vi "Inverter Process Core.vi"() -> ()   [LabVIEW 2019, in "Main.lvclass"]
uses:
  Main.lvclass
  DataTypes/PrivateAsynEv_Main--enum.ctl
  Common/DataTypes/Measurement Config--cluster.ctl
  Common/DataTypes/Acquisition Mode--cluster.ctl
  Common/DataTypes/DAQState--enum.ctl
  Common/DataTypes/LogState--enum.ctl
  Common/DataTypes/TDMSState--enum.ctl
  DataTypes/ProcessingState--enum.ctl
  Common/DataTypes/inverter offset range--cluster.ctl
  Common/DataTypes/inverter gain range--cluster.ctl
  Common/DataTypes/inverter info v2--cluster.ctl
  Common/DataTypes/Inverter database record v2--cluster.ctl
  support/Data Algorithms/subvis/DataTypes/ESR alarm variables.ctl
  support/Data Algorithms/subvis/DataTypes/averaging variables.ctl
  support/Data Algorithms/subvis/DataTypes/Processing loop variables--cluster.ctl
  Common/DataTypes/RawChannelData--cluster.ctl
  Common/DataTypes/RawDAQData--cluster.ctl
  support/Data Algorithms/subvis/DataTypes/Gain control.ctl
  support/Data Algorithms/subvis/DataTypes/ESR scaling--cluster.ctl
  Common/DataTypes/TD Async CmdMsg EventData--cluster.ctl
  Common/DataTypes/UpdateControlValue EvData--cluster.ctl
  DataTypes/ProcessingStateChg EvData--cluster.ctl
  DataTypes/Public Events--cluster.ctl
  DAQ_Engine/DAQ_Engine.lvclass
  Config/Config.lvclass
  Log_Engine/Log_Engine.lvclass
  DataTypes/Dependency--cluster.ctl
  DataTypes/Settings--cluster.ctl
  Common/DataTypes/RawDAQDataQRef--cluster.ctl
  Common/DataTypes/ChannelWaveforms--cluster.ctl
  Common/DataTypes/InverterWaveforms--cluster.ctl
  Common/DataTypes/InverterWaveforms--QRef.ctl
  DataTypes/DataProcessAuxData--cluster.ctl
  Common/DataTypes/DataProcAuxDat--Qref.ctl
  DataTypes/InverterInfo--cluster.ctl
  DataTypes/Process - AppData--cluster.ctl
panel:
  in  "SM2 AppData":T1={"Core"={"Current VI Reference"=refnum, "Close Panel on Exit?"=FALSE}, "Your Boolean data"=FALSE, "Your string data"="", "SMQ"=refnum, "Initialized?"=FALSE, "Self Reference"=refnum, "Simulation?"=FALSE, "process sync"=refnum, "vData"=variant, "Settings"={"Simulation"=FALSE, "Signal scaling"=[], "ESR scaling"=[], "num readings to average"=[], "ESR alarm threshhold (%)"=[], "UseDummyVrms"=FALSE, "Dummy Vrms"=0.0, "Inverter Database File"=path "", "default Inverter (name)"=[]}, "Dependency"={"Config"=refnum, "DAQ"=refnum, "Log_Engine"=refnum}, "Public Events"={"Main.AsyncCmd Event"=refnum, "Main.AsyncMsg Event"=refnum, "stop process"=refnum, "UpdateControlValue Ev"=refnum, "ProcessingStateChg Ev"=refnum}, "RawDaqDataQ"=refnum, "InverterWaveformsQ"=refnum, "Processing loop variables"={"DUT ESR avg"=[], "DUT  PF avg"=[], "DUT  Power avg "=[], "DUT processed data"=[], "ESR alarm variables"=[], "Status data"=[], "CurrInverter"=[], "miscellaneous"=[], "DUT INVERTER data"=[]}, "Measurement config"={"Data Rate 9775"=3.0, "Data Rate 9215"=1200000.0, "Samples RMS 9215"=480000, "Samples RMS 9775"=3}, "Acquisition mode"=enum."3phase", "DAQState"=enum."Unknown", "Signal scaling"={"Iin ripple gain"=13.333, "Iout ripple gain"=13.333, "Iout 60Hz gain "=14.286, "Vout 60Hz gain "=20.0, "Iin ripple offest"=0.0, "Iout ripple offset"=0.0, "Iout 60Hz offset"=0.0, "Vout 60Hz offset"=0.0}, "PrivateAsync Ev"=refnum, "LogState"=enum."Unknown", "TDMSState"=enum."Unknown", "InvWfmsQ-DT"=refnum, "DPAuxDataQ"=refnum, "ProcessingState"=enum."Idle", "InverterInfo"={"Inverter ID"=""}, "ProcLoopInterval"=0, "StoredESR Baseline"=[], "StoreESR BLine Flag"=FALSE, "UseSavedESR BLine Flag"=FALSE} {"Processing loop variables"."CurrInverter"."last updated" format="%<%H:%M\n%d/%m/%Y>T"; "Processing loop variables"."CurrInverter"."set flag" items=["False", "True"]; "Settings"."Dummy Vrms" format="%.2g"}
  in  "ESR scaling":T4
  in  "UseDummyVrms":bool
  in  "Dummy Vrms":dbl=120.0
  in  "reset averaging":bool
  in  "Signal scaling":T3={"Iin ripple gain"=13.333, "Iout ripple gain"=13.333, "Iout 60Hz gain "=14.286, "Vout 60Hz gain "=20.0, "Iin ripple offest"=0.0, "Iout ripple offset"=0.0, "Iout 60Hz offset"=0.0, "Vout 60Hz offset"=0.0}
  out "DAQ data":T24
  out "RawDaqDataQ size":i32
  in  "sampling rate (Hz)":i32
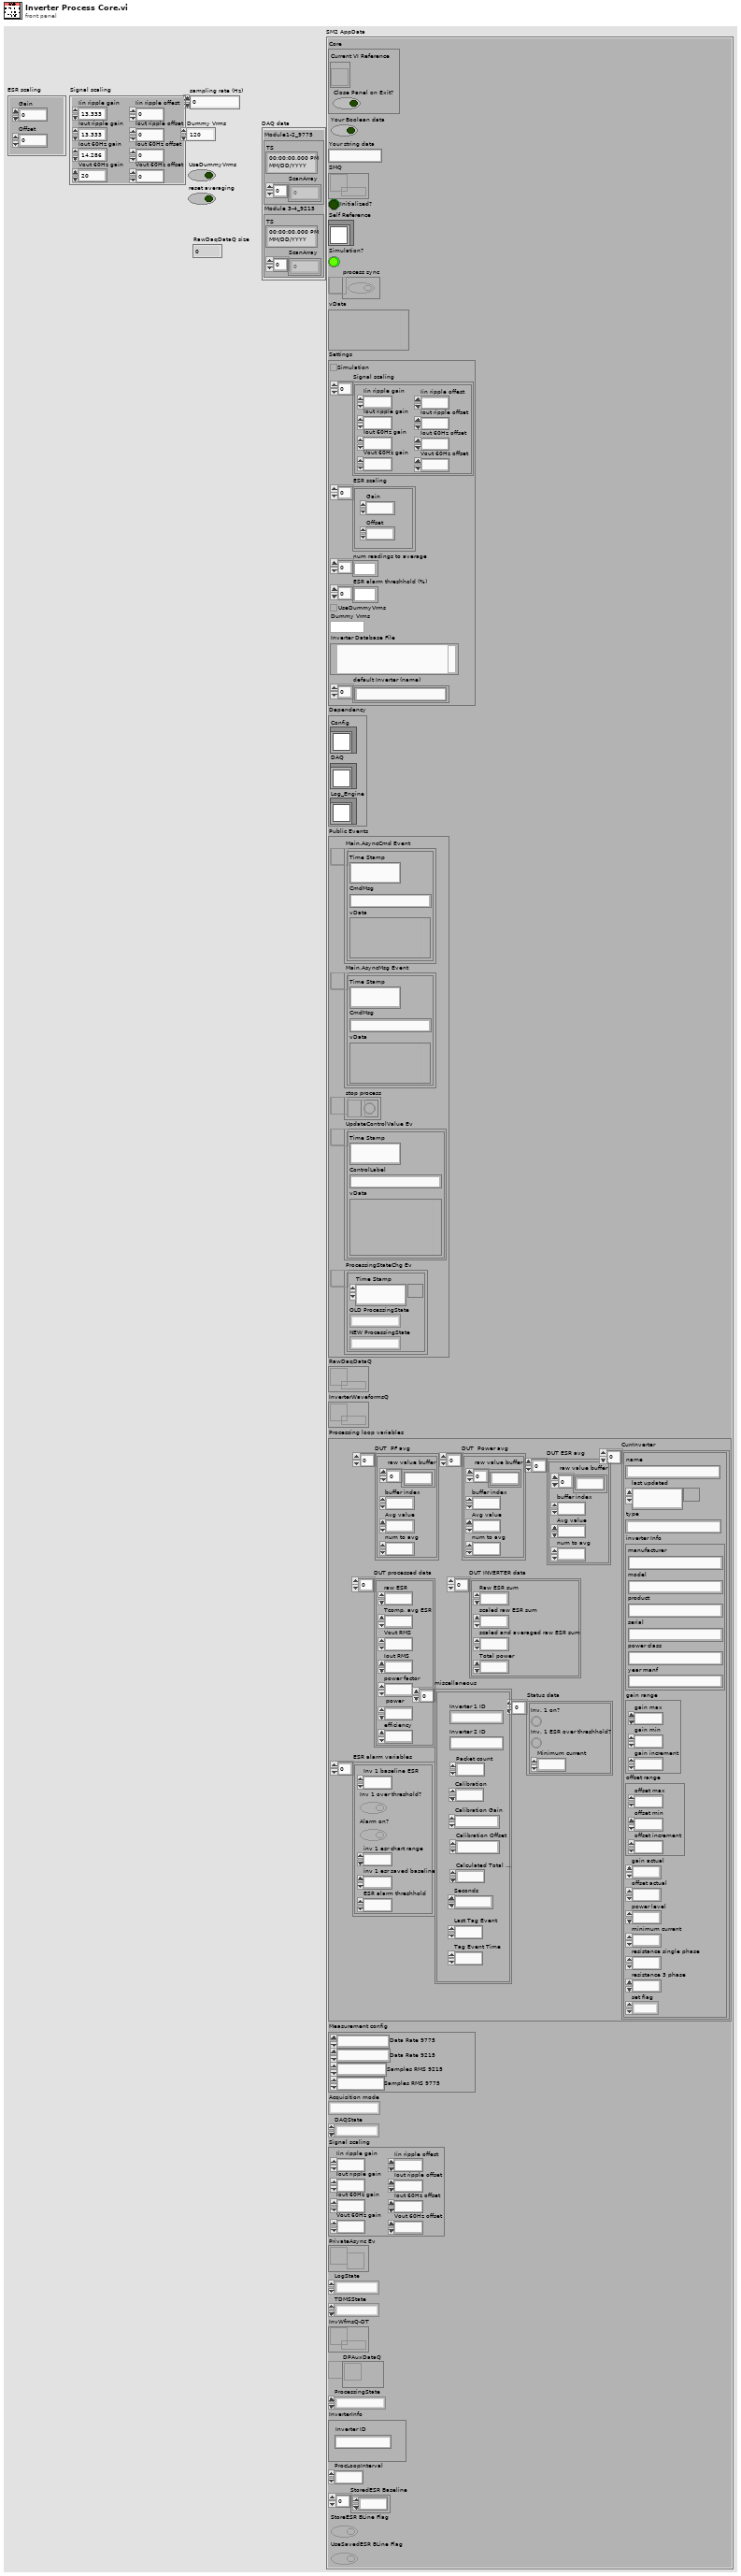
[diagram p1: front panel]
types:
  T1 = typedef "Main.lvclass/Process - AppData--cluster.ctl" = cluster{"Core":cluster{"Current VI Reference":refnum<vi>, "Close Panel on Exit?":bool}, "Your Boolean data":bool, "Your string data":string, "SMQ":refnum<queue>, "Initialized?":bool, "Self Reference":refnum<class "Main.lvclass">, "Simulation?":bool, "process sync":refnum<notifier>, "vData":variant, "Settings":T2, "Dependency":T5, "Public Events":T6, "RawDaqDataQ":T7, "InverterWaveformsQ":T8, "Processing loop variables":T9, "Measurement config":T16, "Acquisition mode":T17, "DAQState":T18, "Signal scaling":T3, "PrivateAsync Ev":refnum<user-event>, "LogState":T19, "TDMSState":T20, "InvWfmsQ-DT":T8, "DPAuxDataQ":T21, "ProcessingState":T22, "InverterInfo":T23, "ProcLoopInterval":u32, "StoredESR Baseline":dbl[], "StoreESR BLine Flag":bool, "UseSavedESR BLine Flag":bool}
  T2 = typedef "Main.lvclass/Settings--cluster.ctl" = cluster{"Simulation":bool, "Signal scaling":T3[], "ESR scaling":T4[], "num readings to average":i32[], "ESR alarm threshhold (%)":i32[], "UseDummyVrms":bool, "Dummy Vrms":dbl, "Inverter Database File":path, "default Inverter (name)":string[]}
  T3 = typedef "Main.lvclass/Gain control.ctl" = cluster{"Iin ripple gain":dbl, "Iout ripple gain":dbl, "Iout 60Hz gain ":dbl, "Vout 60Hz gain ":dbl, "Iin ripple offest":dbl, "Iout ripple offset":dbl, "Iout 60Hz offset":dbl, "Vout 60Hz offset":dbl}
  T4 = typedef "Main.lvclass/ESR scaling--cluster.ctl" = cluster{"Gain":dbl, "Offset":dbl}
  T5 = typedef "Main.lvclass/Dependency--cluster.ctl" = cluster{"Config":refnum<class "Config.lvclass">, "DAQ":refnum<class "DAQ_Engine.lvclass">, "Log_Engine":refnum<class "Log_Engine.lvclass">}
  T6 = typedef "Main.lvclass/Public Events--cluster.ctl" = cluster{"Main.AsyncCmd Event":refnum<user-event>, "Main.AsyncMsg Event":refnum<user-event>, "stop process":refnum<user-event>, "UpdateControlValue Ev":refnum<user-event>, "ProcessingStateChg Ev":refnum<user-event>}
  T7 = typedef "RawDAQDataQRef--cluster.ctl" = refnum<queue>
  T8 = typedef "InverterWaveforms--QRef.ctl" = refnum<queue>
  T9 = typedef "Main.lvclass/Processing loop variables--cluster.ctl" = cluster{"DUT ESR avg":T10[], "DUT  PF avg":T10[], "DUT  Power avg ":T10[], "DUT processed data":cluster{"raw ESR":dbl, "Tcomp, avg ESR":dbl, "Vout RMS":dbl, "Iout RMS":dbl, "power factor":dbl, "power":dbl, "efficiency":dbl}[], "ESR alarm variables":T11[], "Status data":cluster{"Inv. 1 on?":bool, "Inv. 1 ESR over threshhold?":bool, "Minimum current":dbl}[], "CurrInverter":T12[], "miscellaneous":cluster{"Inverter 1 ID":string, "Inverter 2 ID":string, "Packet count":u32, "Calibration":dbl, "Calibration Gain":dbl, "Calibration Offset":dbl, "Calculated Total Power":dbl, "Seconds":dbl, "Last Tag Event":dbl, "Tag Event Time":dbl}[], "DUT INVERTER data":cluster{"Raw ESR sum":dbl, "scaled raw ESR sum":dbl, "scaled and averaged raw ESR sum":dbl, "Total power":dbl}[]}
  T10 = typedef "Main.lvclass/averaging variables.ctl" = cluster{"raw value buffer":dbl[], "buffer index":i32, "Avg value":dbl, "num to avg":i32}
  T11 = typedef "Main.lvclass/ESR alarm variables.ctl" = cluster{"Inv 1 baseline ESR":dbl, "Inv 1 over threshold?":bool, "Alarm on?":bool, "inv 1 esr chart range":dbl, "inv 1 esr saved baseline":dbl, "ESR alarm threshhold":dbl}
  T12 = typedef "Inverter database record v2--cluster.ctl" = cluster{"name":string, "last updated":timestamp, "type":string, "inverter Info":T13, "gain range":T14, "offset range":T15, "gain actual":dbl, "offset actual":dbl, "power level":dbl, "minimum current":dbl, "resistance single phase":dbl, "resistance 3 phase":dbl, "set flag":u16}
  T13 = typedef "inverter info v2--cluster.ctl" = cluster{"manufacturer":string, "model":string, "product":string, "serial":string, "power class":string, "year manf":string}
  T14 = typedef "inverter gain range--cluster.ctl" = cluster{"gain max":dbl, "gain min":dbl, "gain increment":dbl}
  T15 = typedef "inverter offset range--cluster.ctl" = cluster{"offset max":dbl, "offset min":dbl, "offset increment":dbl}
  T16 = typedef "Measurement Config--cluster.ctl" = cluster{"Data Rate 9775":dbl, "Data Rate 9215":dbl, "Samples RMS 9215":u32, "Samples RMS 9775":u32}
  T17 = typedef "Acquisition Mode--cluster.ctl" = enum16{"3phase", "Single"}
  T18 = typedef "DAQState--enum.ctl" = enum16{"Unknown", "Stopped", "Running", "Error"}
  T19 = typedef "LogState--enum.ctl" = enum16{"Unknown", "Stopped", "Running", "Error"}
  T20 = typedef "TDMSState--enum.ctl" = enum16{"Unknown", "Stopped", "Running", "Error"}
  T21 = typedef "DataProcAuxDat--Qref.ctl" = refnum<queue>
  T22 = typedef "Main.lvclass/ProcessingState--enum.ctl" = enum16{"Idle", "Starting", "Running", "Done", "Error"}
  T23 = typedef "InverterInfo--cluster.ctl" = cluster{"Inverter ID":string}
  T24 = typedef "RawDAQData--cluster.ctl" = cluster{"Module1-2_9775":T25, "Module 3-4_9215":T25}
  T25 = typedef "RawChannelData--cluster.ctl" = cluster{"TS":timestamp, "ScanArray":dbl[]}
  T26 = enum16{"Event Loop -", "Async Loop -", "DataProc Loop - "}
  T27 = typedef "Main.lvclass/PrivateAsynEv_Main--enum.ctl" = enum16{"PrivMain.UpdateMeasSettings", "PrivMain.UpdateAcqMode", "PrivMain.UpdateDAQState", "PrivMain.UpdateLogState", "PrivMain.UpdateTDMSState", "PrivMain.UpdateProcessingState", "PrivMain.Stop&Terminate", "PrivMain.CurrInverterUpdated", "PrivMain.UpdateStoreUseESRBaseline", "PrivMain.SetUnsetAlarm&ESRBLine", "PrivMain.ResetAveraging"}
  T28 = cluster{"VoltageDyn":dbl, "CurrentDyn":dbl, "MotorV SP":dbl}[]
  T29 = typedef "InverterWaveforms--cluster.ctl" = T30[]
  T30 = typedef "ChannelWaveforms--cluster.ctl" = cluster{"Iin ripple ":waveform(dbl), "Iout ripple ":waveform(dbl), "Iout 60Hz":waveform(dbl), "Vout 60Hz":waveform(dbl)}
  T31 = typedef "DataProcessAuxData--cluster.ctl" = cluster{"Time Stamp":timestamp, "Raw ESR sum":dbl, "Inv 1 ON?":bool, "Average scaled ESR sum":dbl, "Inv 1 over threshold?":bool, "Inv 1 ESR":cluster{"ESR Baseline":dbl, "Alarm threshhold (%)":dbl, "Avg value":dbl}, "Max ESR":dbl}
  T32 = typedef "TD MeasData--cluster.ctl" = cluster{"Timestamp":timestamp, "ESR_Ohm":dbl[], "DUT data":T33[], "DUT INVERTER data":cluster{"Raw ESR sum":dbl, "scaled raw ESR sum":dbl, "scaled and averaged raw ESR sum":dbl, "Total power":dbl}[]}
  T33 = typedef "InverterPhaseData--cluster.ctl" = cluster{"RawESR_Ohm":dbl, "TcompAvgESR_Ohm":dbl, "VoutRMS_V":dbl, "IoutRMS_A":dbl, "PF":dbl, "AvgPF":dbl, "Power_W":dbl, "AvgPower_W":dbl, "efficiency":dbl}
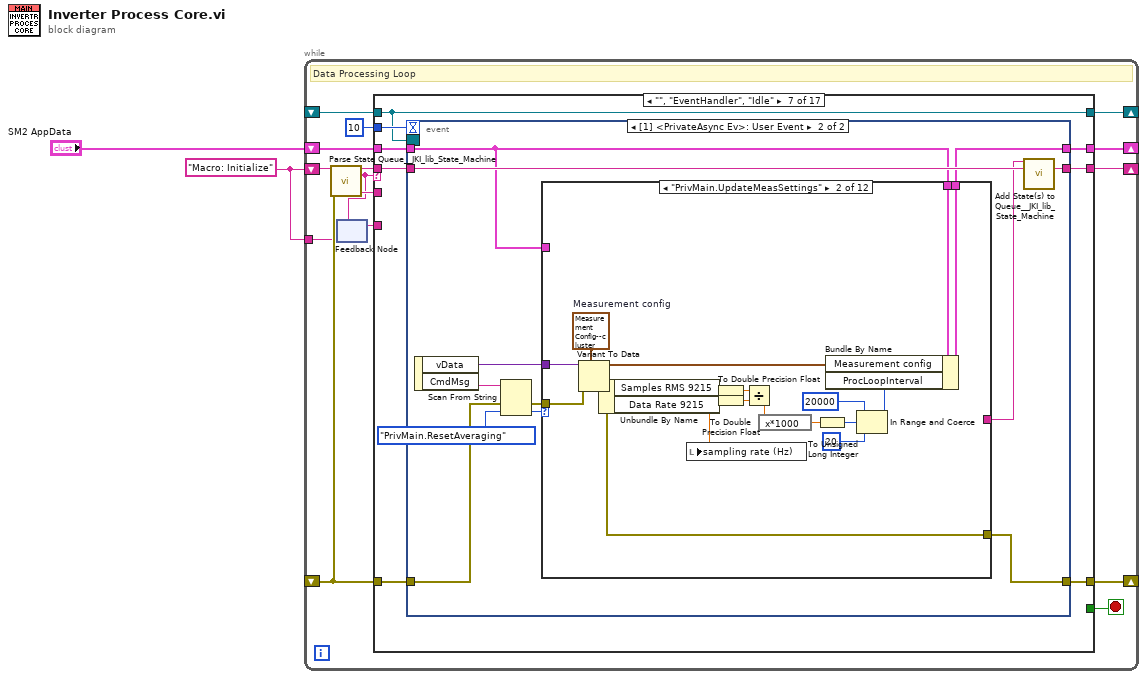
[diagram p0: block diagram]
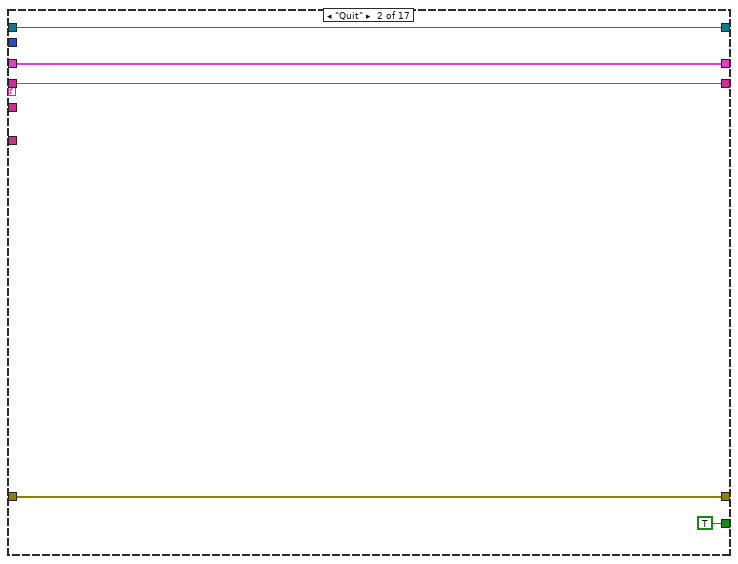
[diagram p3: hidden frame]
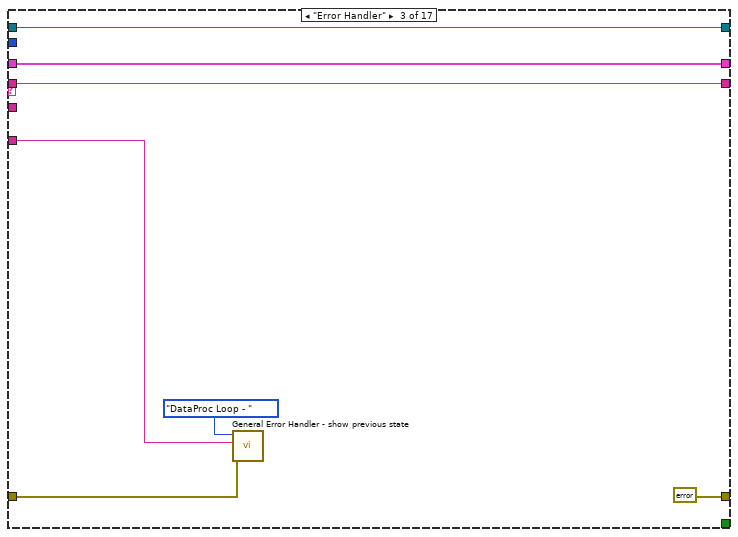
[diagram p4: hidden frame]
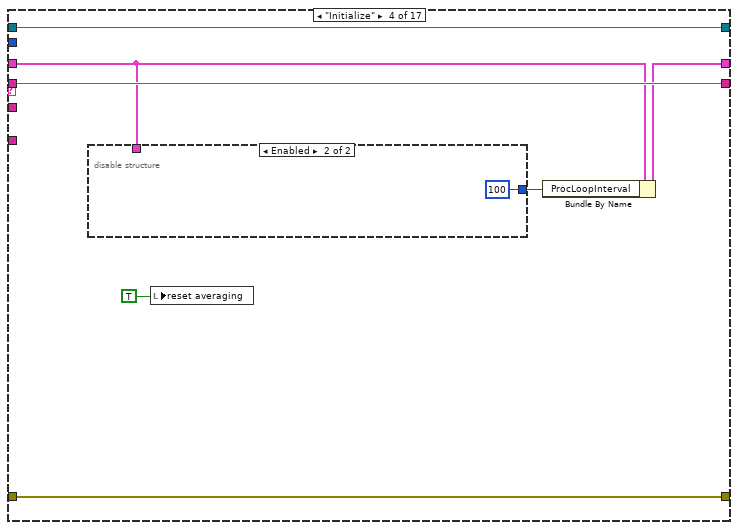
[diagram p5: hidden frame]
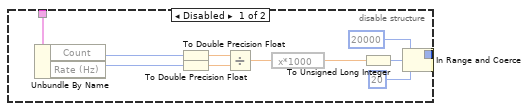
[diagram p6: hidden frame]
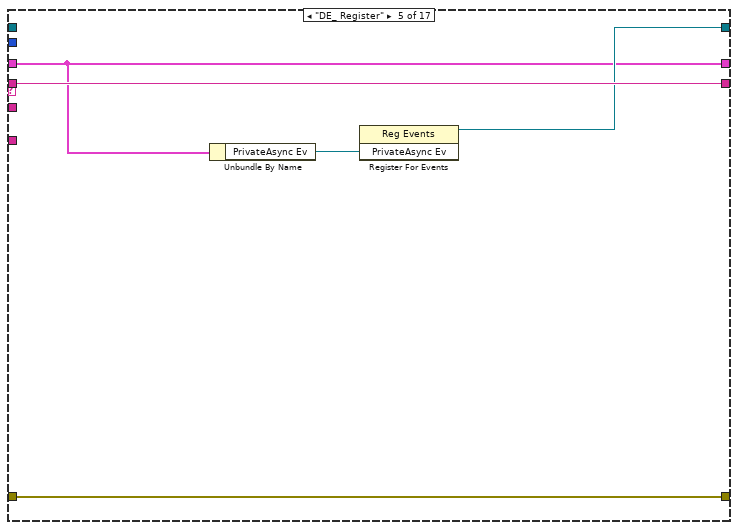
[diagram p7: hidden frame]
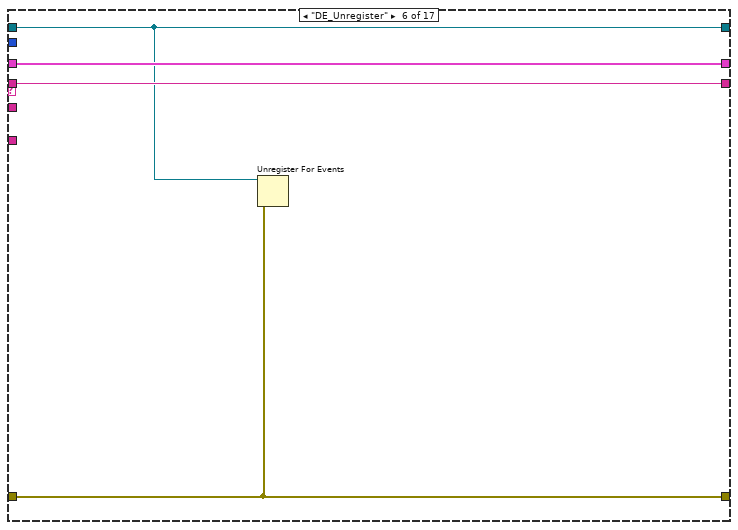
[diagram p8: hidden frame]
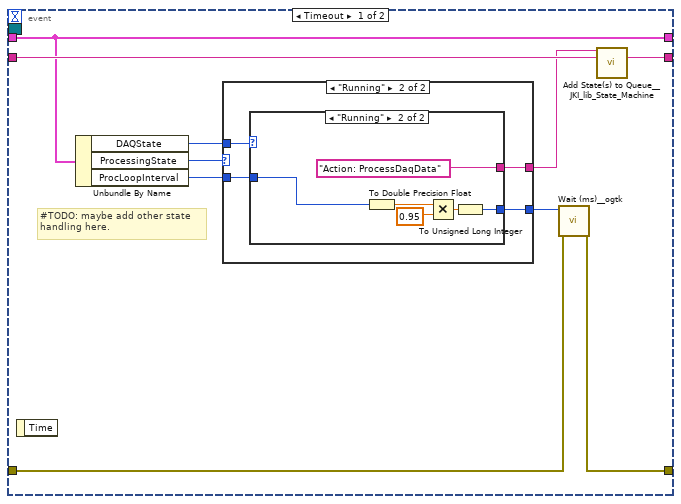
[diagram p9: hidden frame]
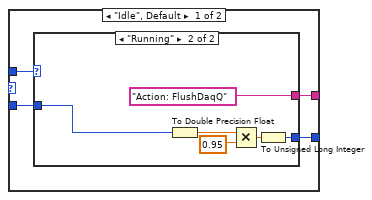
[diagram p10: hidden frame]
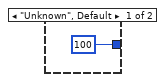
[diagram p11: hidden frame]
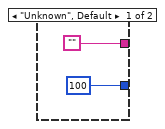
[diagram p12: hidden frame]
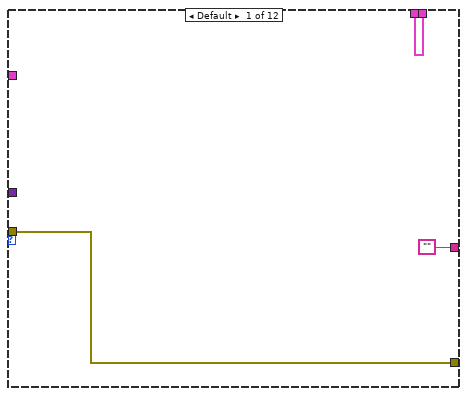
[diagram p13: hidden frame]
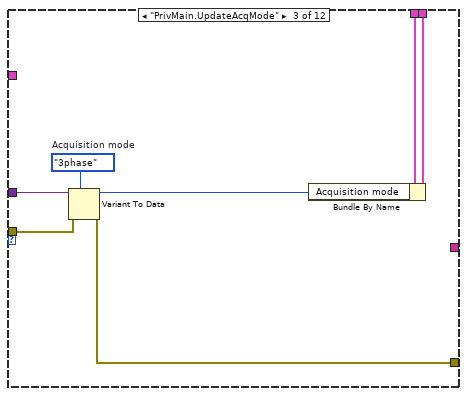
[diagram p14: hidden frame]
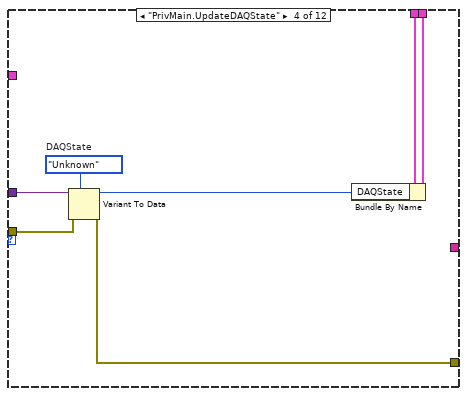
[diagram p15: hidden frame]
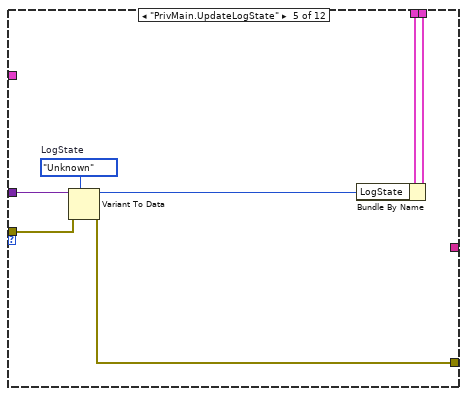
[diagram p16: hidden frame]
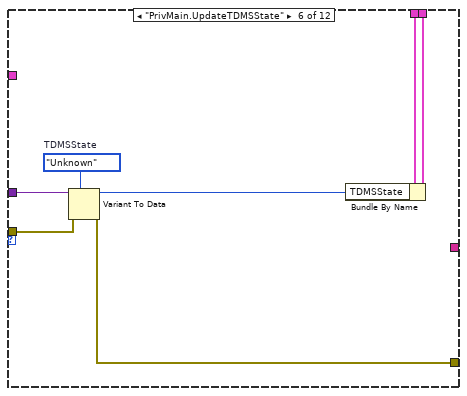
[diagram p17: hidden frame]
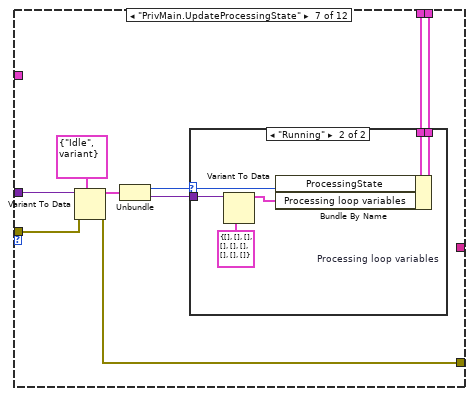
[diagram p18: hidden frame]
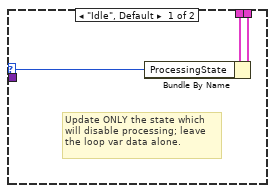
[diagram p19: hidden frame]
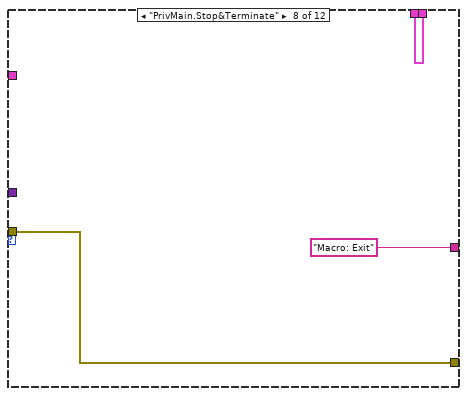
[diagram p20: hidden frame]
diagram:
  w2 = "Macro: Initialize"
  n1 = while {
    shift-right: [w16] -> _
    shift-left: "SM2 AppData" -> [w17]
    shift-right: [w15] -> _
    shift-left: _ -> [w12]
    shift-right: [w10] -> _
    shift-left: w2 -> [w14]
    shift-right: [w8] -> _
    shift-left: _ -> [w7]
    tunnel: w2 -> [w3]
    stop <- w9 stop-if-true
    # "Data Processing Loop"
    n2 = call <vilib>:"Parse State Queue__JKI_lib_State_Machine.vi"("State Queue"=w14, "Error In (no error)"=w12) -> ("Remaining States"=w11:string, "Current State"=w5:string, "Arguments"=w13:string)  [unwired: 11 in]
    n3 = feedback #1(w3) -> (w4:string)
    n4 = feedback-in #1(w5) -> ()
    n5 = case shown="\"\", \"EventHandler\", \"Idle\"" w5 {
      tunnel: w17 -> [w21 w26 w33 w35 w53 w61 w69 w224 w230 w236 w241 w255 w277 w292 w302 w315 w328]
      tunnel: [w21 w26 w33 w36 w53 w61 w68 w224 w230 w236 w241 w244 w277 w293 w303 w315 w333] -> w16
      tunnel: w12 -> [w20 w25 w29 w40 w57 w58 w67 w223 w229 w235 w240 w242 w269 w287 w299 w320 w334]
      tunnel: [w20 w25 errorcluster {"status"=FALSE, "code"=0, "source"=""} ("error constant") w40 w57 w58 w66 w223 w229 w235 w240 w243 w270 w288 w300 w320 w342] -> w15
      tunnel: w13 -> [_ _ _ _ _ _ _ _ _ _ _ _ _ _ _ w316 _]
      tunnel: w11 -> [w19 w24 w32 w38 w56 w60 w65 w222 w226 w232 w237 w258 w284 w298 w311 w319 w356]
      tunnel: [w19 w24 w32 w38 w56 w60 w64 w222 w227 w233 w238 w259 w285 w298 w312 w319 w356] -> w10
      tunnel: [_ TRUE _ _ _ _ _ _ _ _ _ _ _ _ _ _ _] -> w9
      tunnel: [w18 w22 w31 w39 w54 w59 w62 w221 w228 w234 w239 w261 w286 w297 w313 w318 w355] -> w8
      tunnel: w7 -> [w18 w22 w31 w39 _ w59 w62 w221 w228 w234 w239 w261 w286 w297 w313 w318 w355]
      tunnel: 10 -> [_ _ _ _ _ _ w63 _ _ _ _ _ _ _ _ _ _]
      tunnel: w4 -> [_ _ w28 _ _ _ _ _ _ _ _ _ _ _ _ _ _]
      frame Default {
      }
      frame "Quit" {
      }
      frame "Error Handler" {
        n6 = call "General Error Handler - show previous state.vi"("error in (no error)"=w29, "Previous State"=w28, "Loop Select"=T26."DataProc Loop - ") -> ()  [unwired: 7 in, 2 out]
      }
      frame "Initialize" {
        n7 = disable-structure shown="Enabled" {
          disable-tunnel: [w43 u32 100 ("upper limit")] -> w37
          disable-tunnel: w35 -> [w41 _]
          frame Disabled {
            n8 = Unbundle By Name(w41) -> ("Count"=w51:i32, "Rate (Hz)"=w50:i32)
            n9 = To Double Precision Float(number=w51) -> (double precision float=w48:dbl)
            n10 = To Double Precision Float(number=w50) -> (double precision float=w49:dbl)
            n11 = Divide(x=w48, y=w49) -> (x/y=w47:dbl)
            n12 = expression code="x*1000"(w47) -> (w46:dbl)
            n13 = To Unsigned Long Integer(number=w46) -> (unsigned 32bit integer=w45:u32)
            n14 = In Range and Coerce(upper limit=u32 20000, x=w45, lower limit=u32 20) -> (coerced(x)=w43:u32)  [unwired: 1 out]
          }
          frame Enabled {
          }
        }
        n15 = local write "reset averaging"(TRUE) -> ()
        n16 = Bundle By Name(cluster=w35, "ProcLoopInterval"=w37) -> (w36:T1)
      }
      frame "DE_ Register" {
        n17 = Unbundle By Name(w53) -> ("PrivateAsync Ev"=w55:refnum<user-event>)
        n18 = register-events(w55) -> (reference out=w54:refnum<event-registration>)  [unwired: 2 in, 1 out]
      }
      frame "DE_Unregister" {
        n19 = Unregister For Events(event registration refnum=w59, error in=w58) -> ()  [unwired: 1 out]
      }
      frame "", "EventHandler", "Idle" {
        n20 = event shown="[1] <PrivateAsync Ev>: User Event" {
          selector: w62 -> [_ _]
          dyn-events: _ -> [_ _]
          timeout: w63 -> [_ _]
          tunnel: w69 -> [w72 w103]
          tunnel: [w72 w107] -> w68
          tunnel: w67 -> [w73 w105]
          tunnel: [w74 w106] -> w66
          tunnel: w65 -> [w78 w109]
          tunnel: [w79 w108] -> w64
          event Timeout {
            # "#TODO: maybe add other state\nhandling here."
            n21 = event-data() -> ()  [unwired: 1 in, 1 out]
            n22 = Unbundle By Name(w72) -> ("DAQState"=w76:T18, "ProcessingState"=w75:T22, "ProcLoopInterval"=w71:u32)
            n23 = case shown="\"Running\"" w75 {
              tunnel: [w82 w94] -> w77
              tunnel: w76 -> [w83 w93]
              tunnel: w71 -> [w81 w92]
              tunnel: [w80 w91] -> w70
              frame "Idle", Default {
                n24 = case shown="\"Running\"" w83 {
                  tunnel: [_ "Action: FlushDaqQ"] -> w82
                  tunnel: w81 -> [_ w88]
                  tunnel: [u32 100 w85] -> w80
                  frame "Unknown", Default {
                  }
                  frame "Running" {
                    n25 = To Double Precision Float(number=w88) -> (double precision float=w86:dbl)
                    n26 = Multiply(x=w86, y=0.95) -> (x*y=w89:dbl)
                    n27 = To Unsigned Long Integer(number=w89) -> (unsigned 32bit integer=w85:u32)
                  }
                }
              }
              frame "Running" {
                n28 = case shown="\"Running\"" w93 {
                  tunnel: ["" "Action: ProcessDaqData"] -> w94
                  tunnel: w92 -> [_ w98]
                  tunnel: [u32 100 ("ProcLoopInterval") w97] -> w91
                  frame "Unknown", Default {
                  }
                  frame "Running" {
                    n29 = To Double Precision Float(number=w98) -> (double precision float=w99:dbl)
                    n30 = Multiply(x=w99, y=0.95) -> (x*y=w101:dbl)
                    n31 = To Unsigned Long Integer(number=w101) -> (unsigned 32bit integer=w97:u32)
                  }
                }
              }
            }
            n32 = call <userlib>:"Wait (ms)__ogtk.vi"("error in (no error)"=w73, "milliseconds to wait"=w70) -> ("error out"=w74:errorcluster)  [unwired: 8 in, 1 out]
            n33 = call <vilib>:"Add State(s) to Queue__JKI_lib_State_Machine.vi"("State(s) in Front (\"\")"=w77, "State(s) in (\"\")"=w78) -> ("States Out"=w79:string)  [unwired: 13 in]
          }
          event User Event {
            n34 = event-data() -> ("vData"=w110:variant, "CmdMsg"=w114:string)  [unwired: 1 in]
            n35 = Scan From String(input string=w114, error in=w105, default 1=PrivateAsynEv_Main--enum."PrivMain.ResetAveraging" ("PrivAsync")) -> (error out=w111:errorcluster, output 1=w112:T27)  [unwired: 2 in, 2 out]
            n36 = case shown="\"PrivMain.UpdateMeasSettings\"" w112 {
              tunnel: w111 -> [w115 w133 w140 w147 w154 w161 w170 w183 w189 w195 w210 w215]
              tunnel: w110 -> [_ w134 w141 w148 w155 w162 w171 _ w190 _ w211 w216]
              tunnel: w103 -> [w117 w131 w139 w146 w153 w160 w169 w182 w187 w196 w207 w213]
              tunnel: [w117 w130 w138 w145 w152 w159 w168 w182 w186 w194 w206 w213] -> w107
              tunnel: [w115 w129 w136 w143 w150 w157 w167 w183 w188 w191 w209 w214] -> w106
              tunnel: ["" _ _ _ _ _ _ "Macro: Exit" _ _ w203 _] -> w104
              tunnel: w103 -> [_ _ _ _ _ _ _ _ _ w200 _ _]
              frame Default {
              }
              frame "PrivMain.UpdateMeasSettings" {
                w132 = T16 {"Data Rate 9775"=3.0, "Data Rate 9215"=1200000.0, "Samples RMS 9215"=480000, "Samples RMS 9775"=3}  # Measurement config
                n37 = Variant To Data(error in=w133, type=w132, Variant=w134) -> (data=w128:T16, error out=w129:errorcluster)
                n38 = Unbundle By Name(w128) -> ("Samples RMS 9215"=w127:u32, "Data Rate 9215"=w118:dbl)
                n39 = local write "sampling rate (Hz)"(w118) -> ()
                n40 = To Double Precision Float(number=w127) -> (double precision float=w125:dbl)
                n41 = To Double Precision Float(number=w118) -> (double precision float=w126:dbl)
                n42 = Divide(x=w125, y=w126) -> (x/y=w124:dbl)
                n43 = expression code="x*1000"(w124) -> (w123:dbl)
                n44 = To Unsigned Long Integer(number=w123) -> (unsigned 32bit integer=w122:u32)
                n45 = In Range and Coerce(upper limit=u32 20000, x=w122, lower limit=u32 20) -> (coerced(x)=w120:u32)  [unwired: 1 out]
                n46 = Bundle By Name(cluster=w131, "Measurement config"=w128, "ProcLoopInterval"=w120) -> (w130:T1)
              }
              frame "PrivMain.UpdateAcqMode" {
                w135 = Acquisition_Mode--cluster."3phase"  # Acquisition mode
                n47 = Variant To Data(error in=w140, type=w135, Variant=w141) -> (data=w137:T17, error out=w136:errorcluster)
                n48 = Bundle By Name(cluster=w139, "Acquisition mode"=w137) -> (w138:T1)
              }
              frame "PrivMain.UpdateDAQState" {
                w142 = DAQState--enum."Unknown"  # DAQState
                n49 = Variant To Data(error in=w147, type=w142, Variant=w148) -> (data=w144:T18, error out=w143:errorcluster)
                n50 = Bundle By Name(cluster=w146, "DAQState"=w144) -> (w145:T1)
              }
              frame "PrivMain.UpdateLogState" {
                w149 = LogState--enum."Unknown"  # LogState
                n51 = Variant To Data(error in=w154, type=w149, Variant=w155) -> (data=w151:T19, error out=w150:errorcluster)
                n52 = Bundle By Name(cluster=w153, "LogState"=w151) -> (w152:T1)
              }
              frame "PrivMain.UpdateTDMSState" {
                w156 = TDMSState--enum."Unknown"  # TDMSState
                n53 = Variant To Data(error in=w161, type=w156, Variant=w162) -> (data=w158:T20, error out=w157:errorcluster)
                n54 = Bundle By Name(cluster=w160, "TDMSState"=w158) -> (w159:T1)
              }
              frame "PrivMain.UpdateProcessingState" {
                n55 = Variant To Data(error in=w170, type=cluster{"ProcessingState":T22, variant} {"ProcessingState"=enum."Idle", variant}, Variant=w171) -> (data=w165:cluster{"ProcessingState":T22, variant}, error out=w167:errorcluster)
                n56 = Unbundle(w165) -> ("ProcessingState"=w163:T22, w164:variant)
                n57 = case shown="\"Running\"" w163 {
                  selector: w163 -> [w173 w175]
                  tunnel: w169 -> [w174 w180]
                  tunnel: [w172 w179] -> w168
                  tunnel: w164 -> [_ w178]
                  frame "Idle", Default {
                    # "Update ONLY the state which\nwill disable processing; leave\nthe loop var data alone."
                    n58 = Bundle By Name(cluster=w174, "ProcessingState"=w173) -> (w172:T1)
                  }
                  frame "Running" {
                    w177 = T9 {"DUT ESR avg"=[], "DUT  PF avg"=[], "DUT  Power avg "=[], "DUT processed data"=[], "ESR alarm variables"=[], "Status data"=[], "CurrInverter"=[], "miscellaneous"=[], "DUT INVERTER data"=[]}  # Processing loop variables
                    n59 = Variant To Data(type=w177, Variant=w178) -> (data=w176:T9)  [unwired: 1 in, 1 out]
                    n60 = Bundle By Name(cluster=w180, "ProcessingState"=w175, "Processing loop variables"=w176) -> (w179:T1)
                  }
                }
              }
              frame "PrivMain.Stop&Terminate" {
              }
              frame "PrivMain.CurrInverterUpdated" {
                w184 = T12 {"name"="", "last updated"=timestamp(0 s since 1904-01-01), "type"="", "inverter Info"={"manufacturer"="", "model"="", "product"="", "serial"="", "power class"="", "year manf"=""}, "gain range"={"gain max"=0.0, "gain min"=0.0, "gain increment"=0.0}, "offset range"={"offset max"=0.0, "offset min"=0.0, "offset increment"=0.0}, "gain actual"=0.0, "offset actual"=0.0, "power level"=0.0, "minimum current"=0.0, "resistance single phase"=0.0, "resistance 3 phase"=0.0, "set flag"=0}  # CurrInverter
                n61 = Variant To Data(error in=w189, type=w184, Variant=w190) -> (data=w185:T12, error out=w188:errorcluster)
                n62 = Bundle By Name(cluster=w187, "Processing loop variables.CurrInverter"=w185) -> (w186:T1)
              }
              frame "PrivMain.UpdateStoreUseESRBaseline" {
                n63 = Unbundle By Name(w200) -> ("Self Reference"=w199:refnum<class "Main.lvclass">)
                n64 = call "Get StoreESR and UseSavedESR Flag reference.vi"("error in (no error)"=w195, "Main in"=w199) -> ("error out"=w191:errorcluster, "UseSavedESR BLine Ref"=w197:refnum<vi>, "StoreESR BLine Ref"=w198:refnum<vi>)  [unwired: 6 in, 1 out]
                n65 = property class="Bool (strict)"(reference=w198) -> ("Visible"=w193:bool)  [unwired: 1 in, 2 out]
                n66 = property class="Bool (strict)"(reference=w197) -> ("Visible"=w192:bool)  [unwired: 1 in, 2 out]
                n67 = Bundle By Name(cluster=w196, "StoreESR BLine Flag"=w193, "UseSavedESR BLine Flag"=w192) -> (w194:T1)
              }
              frame "PrivMain.SetUnsetAlarm&ESRBLine" {
                n68 = Variant To Data(error in=w210, type=FALSE, Variant=w211) -> (data=w201:bool, error out=w209:errorcluster)
                n69 = Bundle By Name(cluster=w207, "Alarm on?"=w201, "Inv 1 over threshold?"=FALSE) -> (w206:T1)
                n70 = Select(t="Action: Update Alarm & Baseline", s=w201, f="Action: Unset Alarm") -> (s? t:f=w203:string)
              }
              frame "PrivMain.ResetAveraging" {
                n71 = disable-structure shown="Disabled" {
                  disable-tunnel: w216 -> [w219 _]
                  disable-tunnel: w215 -> [w218 w220]
                  disable-tunnel: [w217 w220] -> w214
                  frame Disabled {
                    n72 = Variant To Data(error in=w218, Variant=w219) -> (error out=w217:errorcluster)  [unwired: 1 in, 1 out]
                  }
                  frame Enabled {
                  }
                }
                n73 = local write "reset averaging"(TRUE) -> ()
              }
            }
            n74 = call <vilib>:"Add State(s) to Queue__JKI_lib_State_Machine.vi"("State(s) in Front (\"\")"=w104, "State(s) in (\"\")"=w109) -> ("States Out"=w108:string)  [unwired: 13 in]
          }
        }
      }
      frame "---------- Macro ----------" {
      }
      frame "Macro: Initialize" {
        n75 = call <vilib>:"Add State(s) to Queue__JKI_lib_State_Machine.vi"("State(s) in Front (\"\")"="Initialize\nDE_ Register", "State(s) in (\"\")"=w226) -> ("States Out"=w227:string)  [unwired: 13 in]
      }
      frame "Macro: Exit" {
        n76 = call <vilib>:"Add State(s) to Queue__JKI_lib_State_Machine.vi"("State(s) in Front (\"\")"="DE_Unregister\nAction: FlushDaqQ >> FlushAll\nQuit", "State(s) in (\"\")"=w232) -> ("States Out"=w233:string)  [unwired: 13 in]
      }
      frame "---------- Action ----------" {
        n77 = call <vilib>:"Add State(s) to Queue__JKI_lib_State_Machine.vi"("State(s) in (\"\")"=w237) -> ("States Out"=w238:string)  [unwired: 14 in]
      }
      frame "Action: Update Alarm & Baseline" {
        n78 = Unbundle By Name(w255) -> ("StoreESR BLine Flag"=w254:bool, "StoredESR Baseline"=w253:dbl[], "UseSavedESR BLine Flag"=w256:bool, "scaled and averaged raw ESR sum"=w252:dbl)
        n79 = Unbundle By Name(w255) -> ("Alarm on?"=w246:bool, "Self Reference"=w260:refnum<class "Main.lvclass">)
        n80 = call "Get ESR Chart reference.vi"("error in (no error)"=w242, "Main in"=w260) -> ("error out"=w249:errorcluster, "ESR Chart Ref"=w250:refnum<vi>[])  [unwired: 7 in, 1 out]
        n81 = property class="WFChart (strict)"(reference=w250, error in=w249) -> (error out=w243:errorcluster, "YScale.Maximum"=w248:dbl)  [unwired: 1 out]
        n82 = Select(t=w253, s=w256, f=w252) -> (s? t:f=w247:dbl[])
        n83 = Select(t=w252, s=w254, f=w253) -> (s? t:f=w251:dbl)
        n84 = Bundle By Name(cluster=w255, "StoredESR Baseline"=w251) -> (w245:T1)
        n85 = case shown="False" w246 {
          tunnel: w248 -> [_ w268]
          tunnel: w247 -> [w264 w267]
          tunnel: w245 -> [w263 w266]
          tunnel: [w262 w265] -> w244
          frame True {
            n86 = Bundle By Name(cluster=w263, "Inv 1 baseline ESR"=w264) -> (w262:T1)
          }
          frame False {
            n87 = Bundle By Name(cluster=w266, "Inv 1 baseline ESR"=w267, "inv 1 esr chart range"=w268) -> (w265:T1)
          }
        }
        n88 = call <vilib>:"Add State(s) to Queue__JKI_lib_State_Machine.vi"("State(s) in Front (\"\")"="Action: Update ESR Chart Properties\nAction: Reset ESR BLine Flags" ("State(s) in Front (\"\")"), "State(s) in (\"\")"=w258) -> ("States Out"=w259:string)  [unwired: 13 in]
      }
      frame "Action: Update ESR Chart Properties" {
        n89 = Unbundle By Name(w277) -> ("StoredESR Baseline"=w281:dbl[], "UseSavedESR BLine Flag"=w282:bool, "scaled and averaged raw ESR sum"=w280:dbl)
        n90 = Unbundle By Name(w277) -> ("Self Reference"=w283:refnum<class "Main.lvclass">)
        n91 = call "Get ESR Chart reference.vi"("error in (no error)"=w269, "Main in"=w283) -> ("error out"=w278:errorcluster, "ESR Chart Ref"=w279:refnum<vi>[])  [unwired: 7 in, 1 out]
        n92 = Select(t=w281, s=w282, f=w280) -> (s? t:f=w276:dbl[])
        n93 = Multiply(x=w276, y=4.0) -> (x*y=w274:dbl[])
        n94 = call <vilib>:"Add State(s) to Queue__JKI_lib_State_Machine.vi"("State(s) in (\"\")"=w284) -> ("States Out"=w285:string)  [unwired: 14 in]
        n95 = property class="WFChart (strict)"(reference=w279, error in=w278, "YScale.FormatString"="%.3e", "YScale.Maximum"=w274, "YScale.Minimum"=0.0 ("Y Scale.Range:Minimum"), "History Data"=T28 []) -> (error out=w270:errorcluster)  [unwired: 1 out]
      }
      frame "Action: Reset ESR BLine Flags" {
        w289 = FALSE ("Value")
        n96 = Unbundle By Name(w292) -> ("Self Reference"=w294:refnum<class "Main.lvclass">)
        n97 = call "Get StoreESR and UseSavedESR Flag reference.vi"("error in (no error)"=w287, "Main in"=w294) -> ("error out"=w291:errorcluster, "UseSavedESR BLine Ref"=w295:refnum<vi>, "StoreESR BLine Ref"=w296:refnum<vi>)  [unwired: 6 in, 1 out]
        n98 = property class="Bool (strict)"(reference=w295, error in=w291, "Value"=w289) -> (error out=w290:errorcluster)  [unwired: 1 out]
        n99 = property class="Bool (strict)"(reference=w296, error in=w290, "Value"=w289) -> (error out=w288:errorcluster)  [unwired: 1 out]
        n100 = Bundle By Name(cluster=w292, "StoreESR BLine Flag"=w289, "UseSavedESR BLine Flag"=w289) -> (w293:T1)
      }
      frame "Action: Unset Alarm" {
        w301 = FALSE
        n101 = Unbundle By Name(w302) -> ("inv 1 esr chart range"=w304:dbl)
        n102 = Unbundle By Name(w302) -> ("Self Reference"=w310:refnum<class "Main.lvclass">)
        n103 = call "Get ESR Chart reference.vi"("error in (no error)"=w299, "Main in"=w310) -> ("error out"=w308:errorcluster, "ESR Chart Ref"=w309:refnum<vi>[])  [unwired: 7 in, 1 out]
        n104 = property class="WFChart (strict)"(reference=w309, error in=w308, "YScale.FormatString"="%#_g", "YScale.Maximum"=w304, "YScale.Minimum"=0.0 ("Y Scale.Range:Minimum"), "History Data"=T28 []) -> (error out=w300:errorcluster)  [unwired: 1 out]
        n105 = call <vilib>:"Add State(s) to Queue__JKI_lib_State_Machine.vi"("State(s) in (\"\")"=w311) -> ("States Out"=w312:string)  [unwired: 14 in]
        n106 = Bundle By Name(cluster=w302, "Alarm on?"=w301, "Inv 1 over threshold?"=w301) -> (w303:T1)
      }
      frame "Action: FlushDaqQ" {
        n107 = Unbundle By Name(w315) -> ("RawDaqDataQ"=w317:T7)
        n108 = Flush Queue(queue=w317) -> (error out=w314:errorcluster)  [unwired: 1 in, 2 out]
        n109 = case shown="\"False\", Default" w316 {
          tunnel: w315 -> [_ w324]
          tunnel: w314 -> [_ _]
          frame "False", Default {
          }
          frame "FlushAll" {
            n110 = Unbundle By Name(w324) -> ("InverterWaveformsQ"=w321:T8, "InvWfmsQ-DT"=w322:T8, "DPAuxDataQ"=w323:T21)
            n111 = Flush Queue(queue=w323) -> ()  [unwired: 1 in, 3 out]
            n112 = Flush Queue(queue=w322) -> ()  [unwired: 1 in, 3 out]
            n113 = Flush Queue(queue=w321) -> ()  [unwired: 1 in, 3 out]
          }
        }
      }
      frame "Action: ProcessDaqData" {
        n114 = Unbundle By Name(w328) -> ("InvWfmsQ-DT"=w343:T8, "DPAuxDataQ"=w344:T21, "InverterWaveformsQ"=w345:T8)
        n115 = Unbundle By Name(w328) -> ("TDMSState"=w347:T20)
        n116 = Unbundle By Name(w328) -> ("Acquisition mode"=w326:T17, "Processing loop variables"=w352:T9, "RawDaqDataQ"=w325:T7)
        n117 = Unbundle By Name(w328) -> ("LogState"=w329:T19)
        n118 = Not Equal?(x=w347, y=TDMSState--enum."Running") -> (x != y?=w340:bool)
        n119 = Not Equal?(x=w329, y=LogState--enum."Running") -> (x != y?=w327:bool)
        n120 = Get Queue Status(queue=w325, error in (no error)=w334) -> (queue out=w338:T7, error out=w335:errorcluster, # elements in queue=→"RawDaqDataQ size":i32)  [unwired: 1 in, 5 out]
        n121 = Dequeue Element(queue=w338, timeout in ms (-1)=8000, error in (no error)=w335) -> (element=w353:T24, timed out?=w337:bool, error out=w354:errorcluster)  [unwired: 1 out]
        n122 = case shown="False" w337 {
          tunnel: w354 -> [w373 w390]
          tunnel: w353 -> [w368 _]
          tunnel: w352 -> [w370 w389]
          tunnel: "sampling rate (Hz)" -> [w371 _]
          tunnel: "ESR scaling" -> [w367 _]
          tunnel: "UseDummyVrms" -> [w366 _]
          tunnel: "Dummy Vrms" -> [w365 _]
          tunnel: "reset averaging" -> [w359 _]
          tunnel: w345 -> [w380 _]
          tunnel: w344 -> [w379 _]
          tunnel: w343 -> [w377 _]
          tunnel: [w375 w390] -> w342
          tunnel: "Signal scaling" -> [w369 _]
          tunnel: w340 -> [w362 _]
          tunnel: [w361 w389] -> w332
          tunnel: w327 -> [w360 _]
          tunnel: w326 -> [w357 _]
          frame False {
            w383 = FALSE  # UpdateTS (T)
            n123 = call "Process DAQ Data.vi"("reset averaging"=w359, "Processing loop variables"=w370, "RawDAQData in"=w368, "Signal scaling"=w369, "error in"=w373, "Data Rate 9215 (S/s)"=w371, "ESR scaling"=w367, "Acquisition mode"=w357, "Use dummy Vout?"=w366, "Dummy Vrms"=w365) -> ("InverterWaveforms"=w363:T29, "Processing loop vars out"=w361:T9, "DataProcAuxData"=w358:T31[], "MeasData"=w364:T32, "error out"=w372:errorcluster)  [unwired: 5 in]
            n124 = case shown="False" w362 {
              tunnel: w380 -> [w387 _]
              tunnel: [w386 errorcluster {"status"=FALSE, "code"=0, "source"=""} ("error constant")] -> w378
              tunnel: w363 -> [w385 _]
              frame False {
                n125 = Enqueue Element(queue=w387, element=w385) -> (error out=w386:errorcluster)  [unwired: 2 in, 2 out]
              }
              frame True {
              }
            }
            n126 = case shown="True" w359 {
              frame False {
              }
              frame True {
                n127 = local write "reset averaging"(FALSE) -> ()
              }
            }
            n128 = call "Set MeasData in Q.vi"("UpdateTS (T)"=w383, "error in (no error)"=w372, "MeasData out"=w364) -> ("error out"=w382:errorcluster)  [unwired: 7 in, 1 out]
            n129 = Enqueue Element(queue=w379, element=w358, error in (no error)=w378) -> (error out=w376:errorcluster)  [unwired: 1 in, 2 out]
            n130 = call "Get MeasData Q and Insert Logging Data.vi"("error in"=w382, "bypass"=w360) -> ("error out"=w381:errorcluster)  [unwired: 6 in, 2 out]
            n131 = Enqueue Element(queue=w377, element=w363, error in (no error)=w376) -> (error out=w374:errorcluster)  [unwired: 1 in, 2 out]
            n132 = Merge Errors(w374, w381) -> (w375:errorcluster)
            "DAQ data" <- w368
          }
          frame True {
          }
        }
        n133 = Bundle By Name(cluster=w328, "Processing loop variables"=w332) -> (w333:T1)
      }
    }
  }
